vi "X-Axis_Generator_x.vi"(0 "Central Wavelength":dbl=600.0 format="%.2f", 2 "Current Grating Density":T3=enum."600" caption="Grating Density", 5 "X-Axis Unit":T2=enum."nm", 7 "Current Detector":T1, 8 "X-Axis Points":enum16{"1024", "512", "3"}(ring)) -> (12 "X-axis  (nm)":dbl[](array[numeric])=[571.2504622529284, 585.6489231225254, 600.0000000000001, 614.300024178551, 628.5453659653462] format="%.4f", 13 "X-axis":dbl[](array[numeric])=[571.2504622529284, 585.6489231225254, 600.0000000000001, 614.300024178551, 628.5453659653462] format="%.4f", 14 "nm (Max)":dbl=628.5453659653462 format="%.4f", 15 "nm (Min)":dbl=571.2504622529284 format="%.4f", 16 "cm-1 (Max)":dbl=17505.45629418217 format="%.2f", 17 "cm-1 (Min)":dbl=15909.750578848963 format="%.2f", 18 "meV (Max)":dbl=2170.4007572687524 format="%.2f", 19 "meV (Min)":dbl=1972.5583911666886 format="%.2f")   [LabVIEW 2021]
doc: "Generate CCD X-array.\nInput can be either from the fileInfo Cluster or from the individual components."
uses:
  Globals and TypeDefs/Type Definitions.llb/McPherson Grating Density.ctl
  Globals and TypeDefs/Type Definitions.llb/Wavelength Unit.ctt
  Globals and TypeDefs/Type Definitions.llb/ListOfDetectors.ctt
  X-Axis Converter.llb/X-Axis Converter.vi
panel:
  out "nm (delta)":dbl=57.29490371241775 format="%.4f"
  out "cm-1 (delta)":dbl=1595.705715333208 format="%.2f"
  out "meV (delta)":dbl=197.8423661020638 format="%.2f"
  out "Detector Pixel Distance":dbl=27.0 format="%.2f"
  out "beta":dbl=0.03851514953863218 format="%.2f"
  out "alpha":dbl=21.141484850461367 format="%.2f"
  out "Spectrometer Mirror angle":dbl=21.18 format="%.2f"
  out "Spectrometer Focal length":dbl=750.0 format="%.1f"
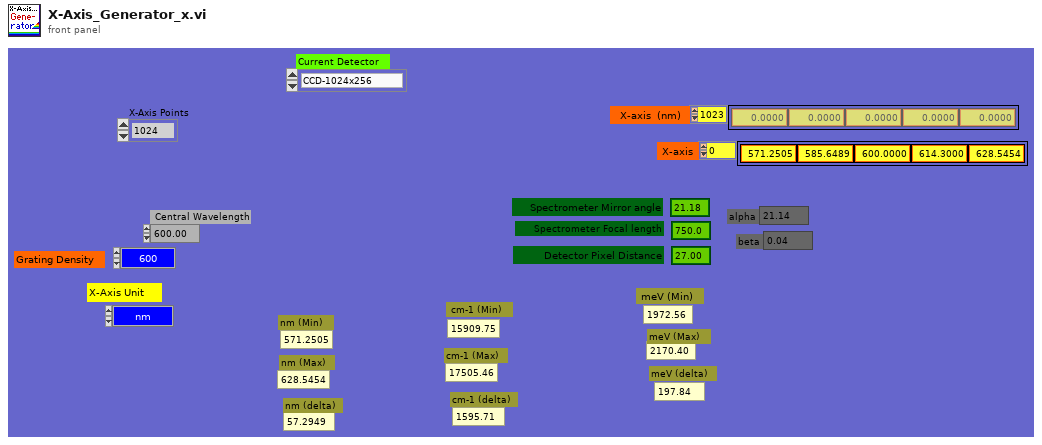
[diagram p1: front panel]
types:
  T1 = typedef "ListOfDetectors.ctt" = enum8{"CCD-1024x256", "InGaAs PDA-1024x1", "CCD-1340x400", "Ge Single Channel", "Si Single Channel", "PMT Single Channel"}
  T2 = typedef "Wavelength Unit.ctt" = enum8{"Point", "nm", "eV", "meV", "cm_1"}
  T3 = typedef "McPherson Grating Density.ctl" = enum8{"150", "300", "600", "1200", "1800"}
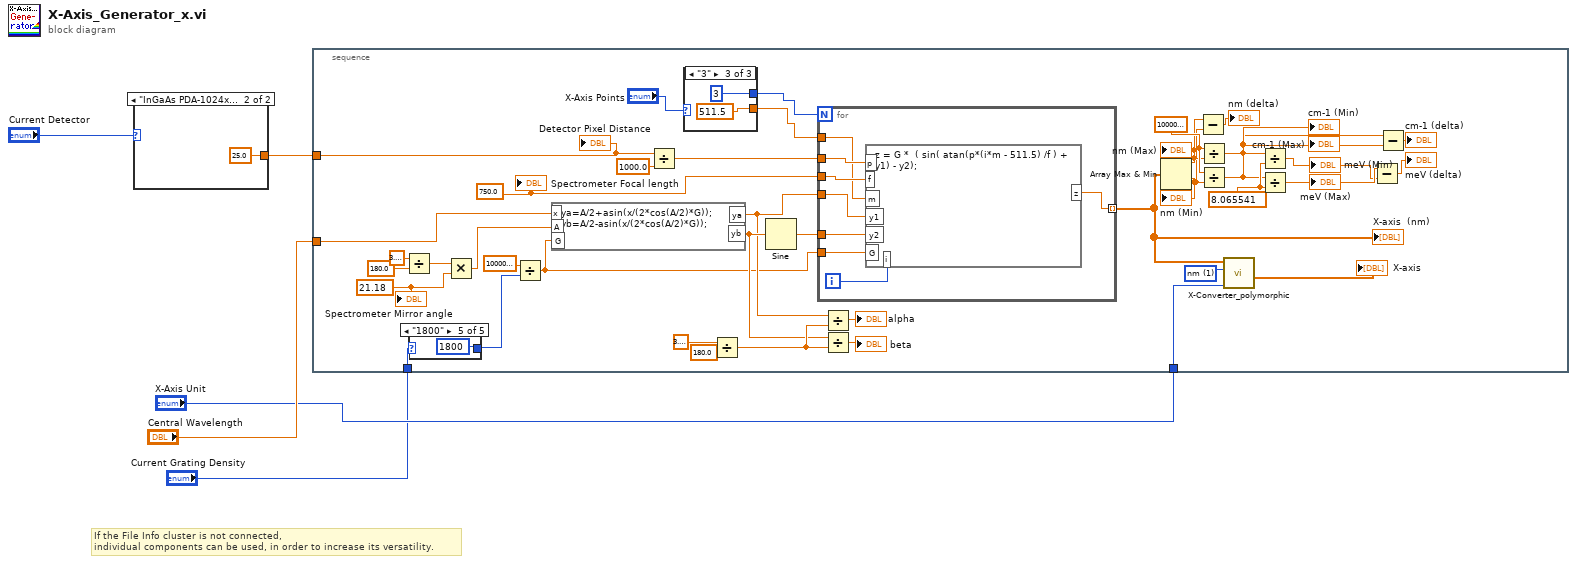
[diagram p0: block diagram]
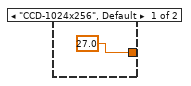
[diagram p2: hidden frame]
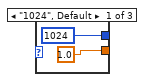
[diagram p3: hidden frame]
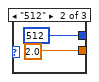
[diagram p4: hidden frame]
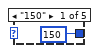
[diagram p5: hidden frame]
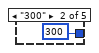
[diagram p6: hidden frame]
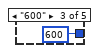
[diagram p7: hidden frame]
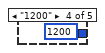
[diagram p8: hidden frame]
diagram:
  # "If the File Info cluster is not connected,\nindividual components can be used, in order to increase its versatility."
  n1 = case shown="\"InGaAs PDA-1024x1\"" "Current Detector" {
    tunnel: [27.0 ("x") 25.0 ("x")] -> w2
    frame "CCD-1024x256", Default {
    }
    frame "InGaAs PDA-1024x1" {
    }
  }
  n2 = stacked-sequence {
    tunnel: "Current Grating Density" -> [w20]
    tunnel: "Central Wavelength" -> [w19]
    tunnel: "X-Axis Unit" -> [w18]
    tunnel: w2 -> [w8]
    frame #0 {
      w22 = 1 items=["Point #", "nm", "eV", "meV", "cm-1"] ("Old X-Axis Unit")
      w32 = 21.18 ("Detector Pixel Distance")
      w13 = 750.0 ("Detector Pixel Distance")
      w42 = 8.065541
      w43 = 10000000.0
      n3 = Divide(x=3.141592653589793, y=180.0) -> (x/y=w27:dbl)
      n4 = case shown="\"1800\"" w20 {
        tunnel: [150 300 600 1200 1800] -> w24
        frame "150" {
        }
        frame "300" {
        }
        frame "600" {
        }
        frame "1200" {
        }
        frame "1800" {
        }
      }
      n5 = Multiply(x=w27, y=w32) -> (x*y=w31:dbl)
      n6 = Divide(x=1000000.0, y=w24) -> (x/y=w10:dbl)
      n7 = formula code="ya=A/2+asin(x/(2*cos(A/2)*G));\nyb=A/2-asin(x/(2*cos(A/2)*G));"("x"=w19, "A"=w31, "G"=w10) -> ("ya"=w12:dbl, "yb"=w25:dbl)
      n8 = Divide(x=w8, y=1000.0) -> (x/y=w14:dbl)
      n9 = case shown="\"3\"" "X-Axis Points" {
        tunnel: [1024 512 3] -> w16
        tunnel: [1.0 2.0 511.5] -> w15
        frame "1024", Default {
        }
        frame "512" {
        }
        frame "3" {
        }
      }
      n10 = Divide(x=3.141592653589793, y=180.0) -> (x/y=w30:dbl)
      n11 = Sine(x=w25) -> (sin(x)=w9:dbl)
      n12 = for {
        N: w16 -> [_]
        tunnel: w14 -> [w54]
        tunnel: w13 -> [w53]
        tunnel: w15 -> [w52]
        tunnel: w12 -> [w51]
        tunnel: w9 -> [w50]
        tunnel: w10 -> [w49]
        tunnel: [w48] -> w11 mode=indexing
        i -> [w55]
        n13 = formula code="z = G *  ( sin( atan(p*(i*m - 511.5) /f ) + y1) - y2);"("p"=w54, "f"=w53, "m"=w52, "y1"=w51, "y2"=w50, "G"=w49, "i"=w55) -> ("z"=w48:dbl)
      }
      "X-axis  (nm)" <- w11
      n14 = Divide(x=w12, y=w30) -> (x/y=→"alpha":dbl)
      n15 = Divide(x=w25, y=w30) -> (x/y=→"beta":dbl)
      n16 = Array Max & Min(array=w11) -> (max value=w36:dbl, min value=w35:dbl)  [unwired: 2 out]
      "nm (Max)" <- w36
      "nm (Min)" <- w35
      n17 = Subtract(x=w36, y=w35) -> (x-y=→"nm (delta)":dbl)
      n18 = Divide(x=w43, y=w36) -> (x/y=w40:dbl)
      "cm-1 (Min)" <- w40
      n19 = Divide(x=w43, y=w35) -> (x/y=w39:dbl)
      "cm-1 (Max)" <- w39
      n20 = call-poly "X-Converter_polymorphic.vi"("X-Axis Unit"=w18, "Old X-Axis Unit"=w22, "X-Axis input"=w11) -> ("X-Axis Output"=→"X-axis":dbl[])  [unwired: 2 in, 3 out]
      n21 = Divide(x=w40, y=w42) -> (x/y=w38:dbl)
      "meV (Min)" <- w38
      n22 = Divide(x=w39, y=w42) -> (x/y=w41:dbl)
      "meV (Max)" <- w41
      n23 = Subtract(x=w41, y=w38) -> (x-y=→"meV (delta)":dbl)
      n24 = Subtract(x=w39, y=w40) -> (x-y=→"cm-1 (delta)":dbl)
      "Spectrometer Focal length" <- w13
      "Spectrometer Mirror angle" <- w32
      "Detector Pixel Distance" <- w8
    }
  }
